vi "Read Position.vi"(11 "Particle in":refnum<class "Particle.lvclass">) -> (2 "Position":T1)   [LabVIEW 2020, in "Particle.lvclass"]
uses:
  Particle.lvclass
  Particle/Position.ctl
  Particle.lvclass/Particle.ctl
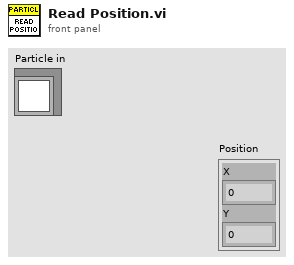
[diagram p1: front panel]
types:
  T1 = typedef "Particle.lvclass/Position.ctl" = cluster{"X":i32, "Y":i32}
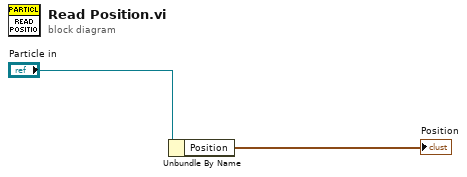
[diagram p0: block diagram]
diagram:
  n1 = Unbundle By Name("Particle in") -> ("Position"=→"Position":T1)
